vi "run.create_begin.vi"(8 "error in":errorcluster, 9 "Time Stamp (Now)":timestamp format="%<%x %.3X>T", 10 "Name":string, 11 "Client in":refnum<class "Client.lvclass">) -> (0 "error out":errorcluster, 2 "RunCreateStaging":refnum<class "RunCreateStaging.lvclass">, 3 "Client out":refnum<class "Client.lvclass">)   [LabVIEW 2020, in "Client.lvclass"]
doc: "Creates a new run in Nominal with a name, start time, and optional description and end time, and returns a handle to it."
uses:
  Client.lvclass
  RunCreateStaging/RunCreateStaging.lvclass
  RunCreateStaging/RunCreateStaging.lvclass/RunCreateStaging.ctl
  Client.lvclass/Client.ctl
  client.lvlib
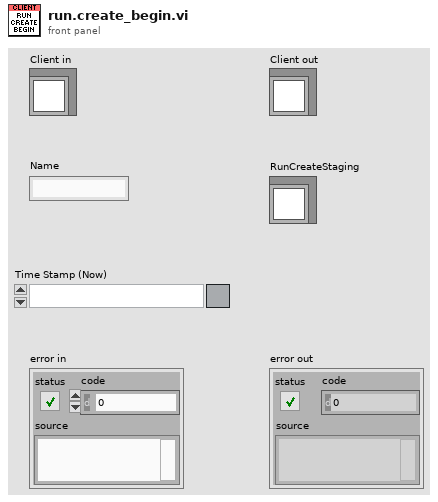
[diagram p1: front panel]
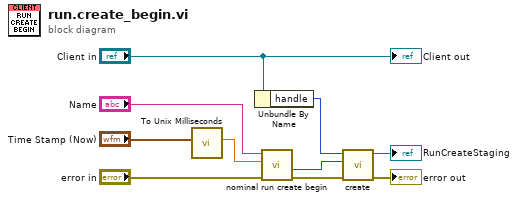
[diagram p0: block diagram]
diagram:
  n1 = call "To Unix Milliseconds.vi"("Time Stamp (Now)"="Time Stamp (Now)") -> ("Unix Milliseconds"=w10:dbl)  [unwired: 10 in]
  n2 = Unbundle By Name("Client in") -> ("handle"=w1:i32)
  n3 = call "nominal run create begin.vi"("error in (no error)"="error in", "start_ms"=w10, "name"="Name") -> ("error out"=w5:errorcluster, "out_staging out"=w6:i32)  [unwired: 6 in, 1 out]
  n4 = call "create.vi"("error in (no error)"=w5, "handle"=w6, "client"=w1) -> ("error out"=→"error out":errorcluster, "RunCreateStaging out"=→"RunCreateStaging":refnum<class "RunCreateStaging.lvclass">)  [unwired: 7 in]
  "Client out" <- "Client in"
